vi "RangeMap3_BM.vi"(0 "InputArray":dbl[][](array[numeric])=array200x200[40000 elements], 5 "distance from origin(cm) X":dbl=51.49398913049394, 7 "angle":dbl=122.5, 9 "probablities":dbl[](array[numeric])=[0.0004688113374269815, 0.0, 2.7006093286747943e-83, 1.1473881061270444e-79, 0.0], 11 "indices":i32[](array[numeric])=[872, 947, 10098, 10125, 10154], 12 "distance from origin(cm) Y":dbl=51.49398913049394) -> (4 "yValues":dbl[](array[numeric])=[35.42357276468377, 34.04136952221157, -134.6058554359637, -135.1034486032537, -135.63790052367628], 8 "OutputArray":dbl[][](array[numeric]), 15 "xValues":dbl[](array[numeric])=[76.71948991817902, 78.88911441253266, 343.6122310502691, 344.39329586823646, 345.2322173393865])   [LabVIEW 2014]
panel:
  out "Anzahl y Elemente":i32
  out "Anzhal x Elemente":i32
  out "Min. Wert":dbl
  out "Max. Wert":dbl=0.08870306401237434
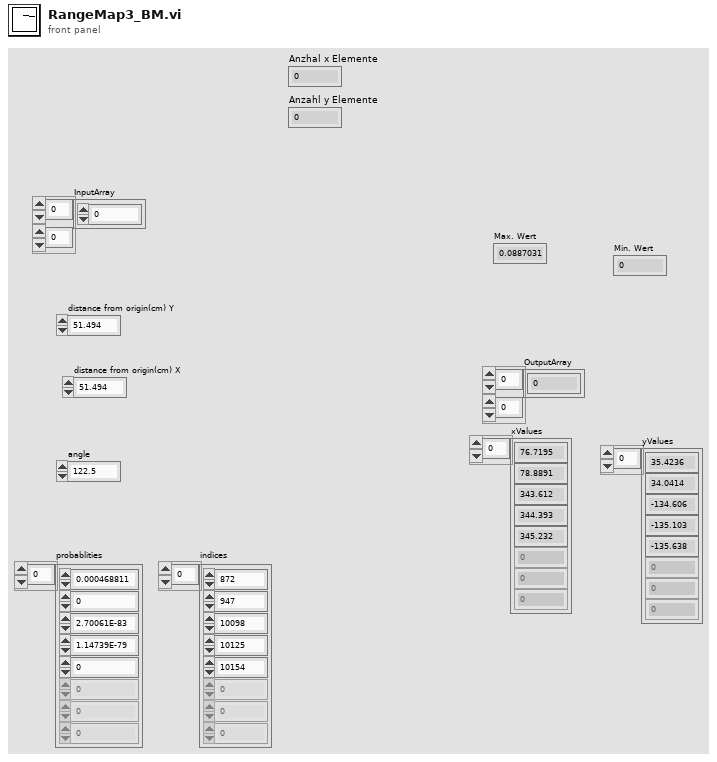
[diagram p1: front panel]
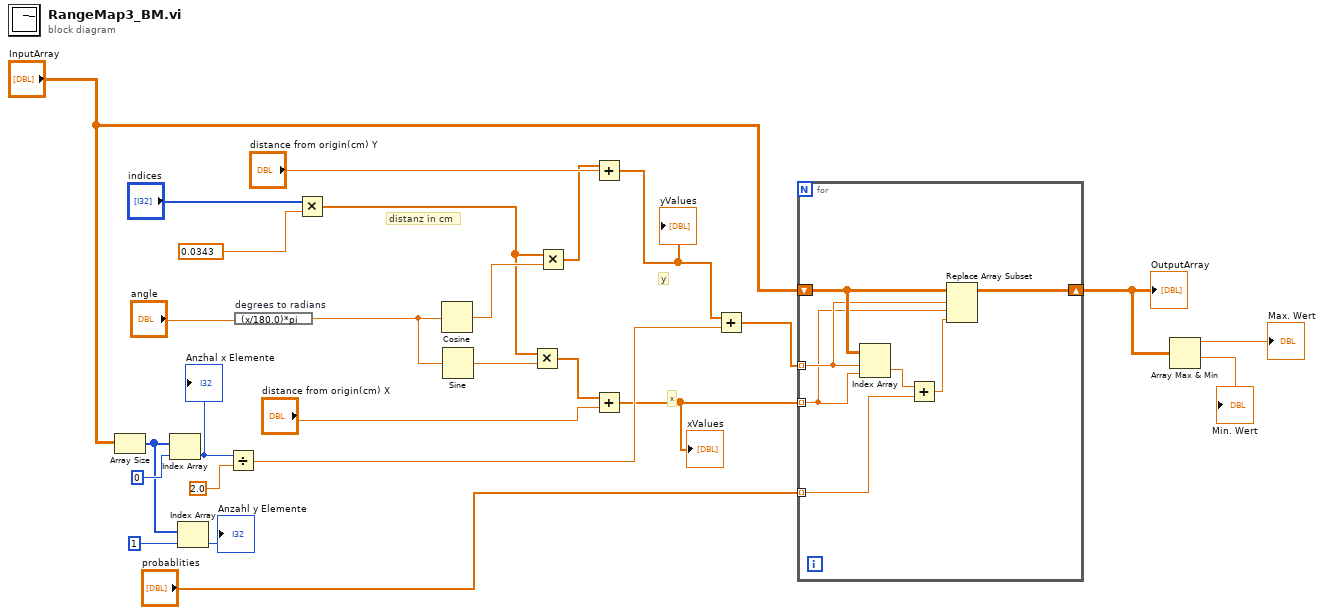
[diagram p0: block diagram]
diagram:
  # "distanz in cm"
  # "y"
  # "x"
  n1 = Array Size(array="InputArray") -> (size(s)=w2:i32[])
  n2 = Index Array(array=w2, index=0) -> (element=w15:i32)
  "Anzhal x Elemente" <- w15
  n3 = Index Array(array=w2, index=1 ("Index")) -> (element=→"Anzahl y Elemente":i32)
  n4 = Divide(x=w15, y=2.0) -> (x/y=w8:dbl)
  n5 = expression code="(x/180.0)*pi" "degrees to radians"("angle") -> (w24:dbl)
  n6 = Multiply(x="indices", y=0.0343) -> (x*y=w22:dbl[])
  n7 = Cosine(x=w24) -> (cos(x)=w25:dbl)
  n8 = Sine(x=w24) -> (sin(x)=w23:dbl)
  n9 = Multiply(x=w22, y=w23) -> (x*y=w18:dbl[])
  n10 = Multiply(x=w22, y=w25) -> (x*y=w6:dbl[])
  n11 = Add(x=w6, y="distance from origin(cm) Y") -> (x+y=w5:dbl[])
  "yValues" <- w5
  n12 = Add(x=w18, y="distance from origin(cm) X") -> (x+y=w4:dbl[])
  "xValues" <- w4
  n13 = Add(x=w5, y=w8) -> (x+y=w19:dbl[])
  n14 = for {
    tunnel: w19 -> [w31] mode=indexing
    tunnel: "probablities" -> [w28] mode=indexing
    shift-right: [w33] -> w13
    shift-left: "InputArray" -> [w32]
    tunnel: w4 -> [w27] mode=indexing
    n15 = Index Array(array=w32, index (row)=w31, index (col)=w27) -> (element=w30:dbl)
    n16 = Add(x=w30, y=w28) -> (x+y=w29:dbl)
    n17 = Replace Array Subset(array=w32, new element=w29, index (row)=w31, index (col)=w27) -> (w33:dbl[][])
  }
  "OutputArray" <- w13
  n18 = Array Max & Min(array=w13) -> (max value=→"Max. Wert":dbl, min value=→"Min. Wert":dbl)  [unwired: 2 out]
